vi "LVClass_HasoData Get Compute Slopes Set - LiftOption.vi"(0 "HasoData in":refnum<class "HasoData.lvclass">, 11 "error in (no error)":errorcluster) -> (4 "HasoData out":refnum<class "HasoData.lvclass">, 13 "lift_algo":bool, 15 "error out":errorcluster)   [LabVIEW 2020, in "HasoData.lvclass"]
doc: "Get LIFT option activation into slopes metadata informations from HasoData object.\n\n<B>HasoDataIn</B> : HasoData object.\n<B>HasoDataOut</B> : HasoData object.\n<B>is_background_removed</B> : Slopes have been calculated with lift option\n<B>ErrorIn </B> : Error\n<B>ErrorOut </B> : Error"
uses:
  HasoData.lvclass
  HasoData.lvclass/HasoData.ctl
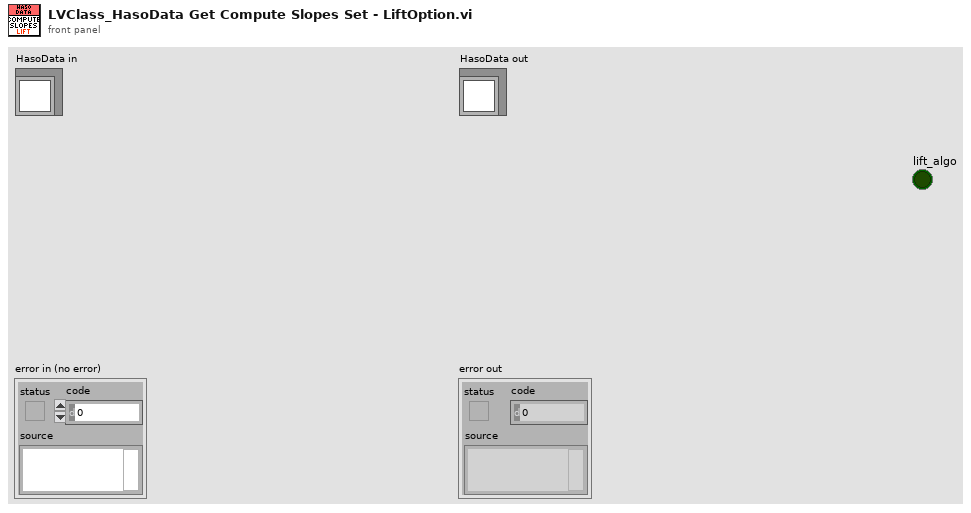
[diagram p1: front panel]
types:
  T1 = typedef "ClassID.ctl" = i64
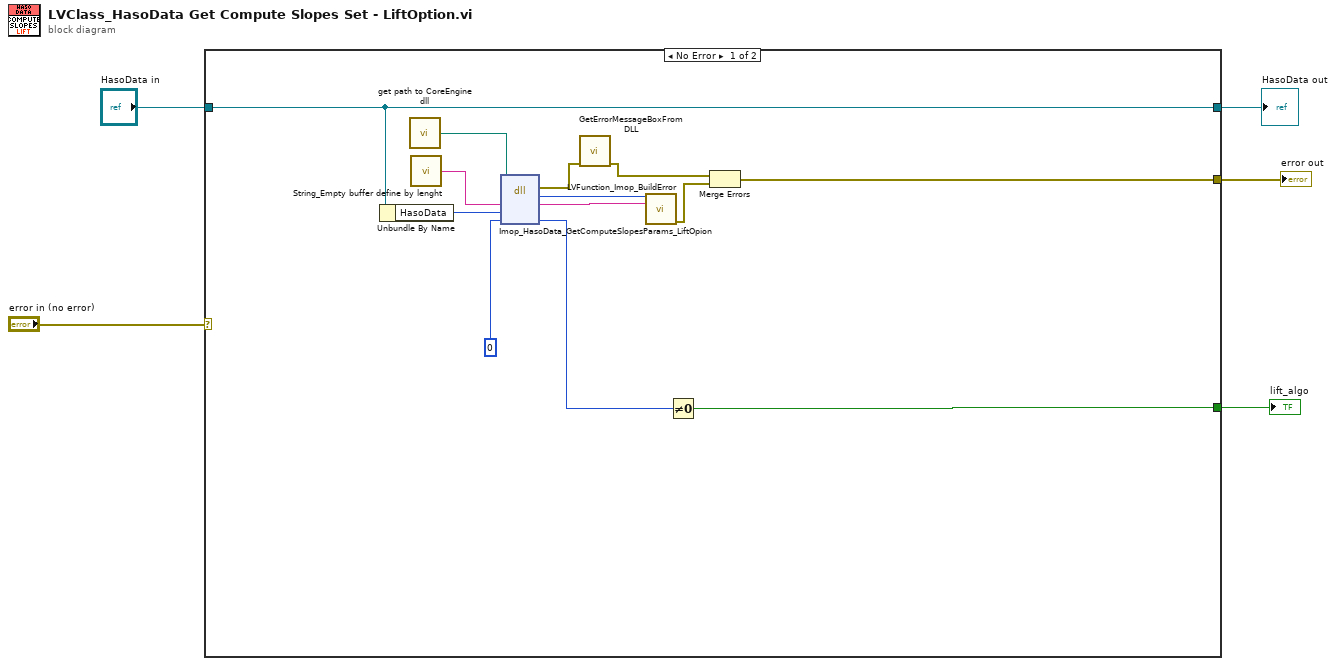
[diagram p0: block diagram]
diagram:
  n1 = case shown="No Error" "error in (no error)" {
    selector: "error in (no error)" -> [_ w20]
    tunnel: [w10 w20] -> w5
    tunnel: [w14 w19] -> w4
    tunnel: "HasoData in" -> [w14 w19]
    tunnel: [w6 _] -> w3
    frame No Error {
      n2 = Unbundle By Name(w14) -> ("HasoData"=w13:T1)
      n3 = call "get path to CoreEngine dll.vi"() -> ("path to wavekit library"=w16:path)  [unwired: 14 in, 1 out]
      n4 = call "String_Empty buffer define by lenght.vi"() -> ("Empty buffer"=w9:string)  [unwired: 1 in]
      n5 = dll-call lib="D:/soft/HASO_v3/SVN_trunk/ImOpCoreEngine4_LV2011/DLLs/c_interface_vc100.dll" fn="Imop_HasoData_GetComputeSlopesParams_LiftOpion"(path in=w16, "message"=w9, "HasoData"=w13, "lift_algo"=u8 0 ("auto_start")) -> (error out=w15:errorcluster, "return type"=w18:i32, "message"=w17:string, "lift_algo"=w7:u8)  [unwired: 3 in, 1 out]
      n6 = call "GetErrorMessageBoxFromDLL.vi"("error IN"=w15) -> ("error OUT"=w12:errorcluster)  [unwired: 10 in]
      n7 = call "LVFunction_Imop_BuildError.vi"("code"=w18, "String to Prepend to source (\"\")"=w17) -> ("error out"=w11:errorcluster)  [unwired: 13 in]
      n8 = Not Equal To 0?(x=w7) -> (x != 0?=w6:bool)
      n9 = Merge Errors(w12, w11) -> (w10:errorcluster)
    }
    frame Error {
    }
  }
  "error out" <- w5
  "HasoData out" <- w4
  "lift_algo" <- w3
